vi "Util - Unbundle - 1Ch.vi"(10 "output":T1) -> (1 "Timed Out?":bool, 2 "DSP Overflow":bool)   [LabVIEW 2015, in "DDC_7976R_v1.lvlib"]
uses:
  DDC_7976R_v1.lvlib
  Typedef - internal -02.ctl
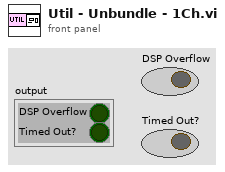
[diagram p1: front panel]
types:
  T1 = typedef "DDC_7976R_v1.lvlib/Typedef - internal -02.ctl" = cluster{"DSP Overflow":bool, "Timed Out?":bool}
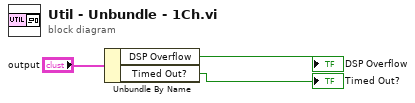
[diagram p0: block diagram]
diagram:
  n1 = Unbundle By Name("output") -> ("DSP Overflow"=→"DSP Overflow":bool, "Timed Out?"=→"Timed Out?":bool)
